vi "Test_Selection.vi"() -> ()   [LabVIEW 2017]
panel:
  out "File Transfer":u8
  in  "Recipe Download msg":string
  out "Exit":bool
  in  "Access Level":string
  out "Text Files":string[](array[string])
  out "Tests":string[](array[string])
  out "Paths":T1
  out "Rights":T2
  in  "Operator":string
  in  "Serial:":string
  in  "Part:":string
  in  "Test:":string
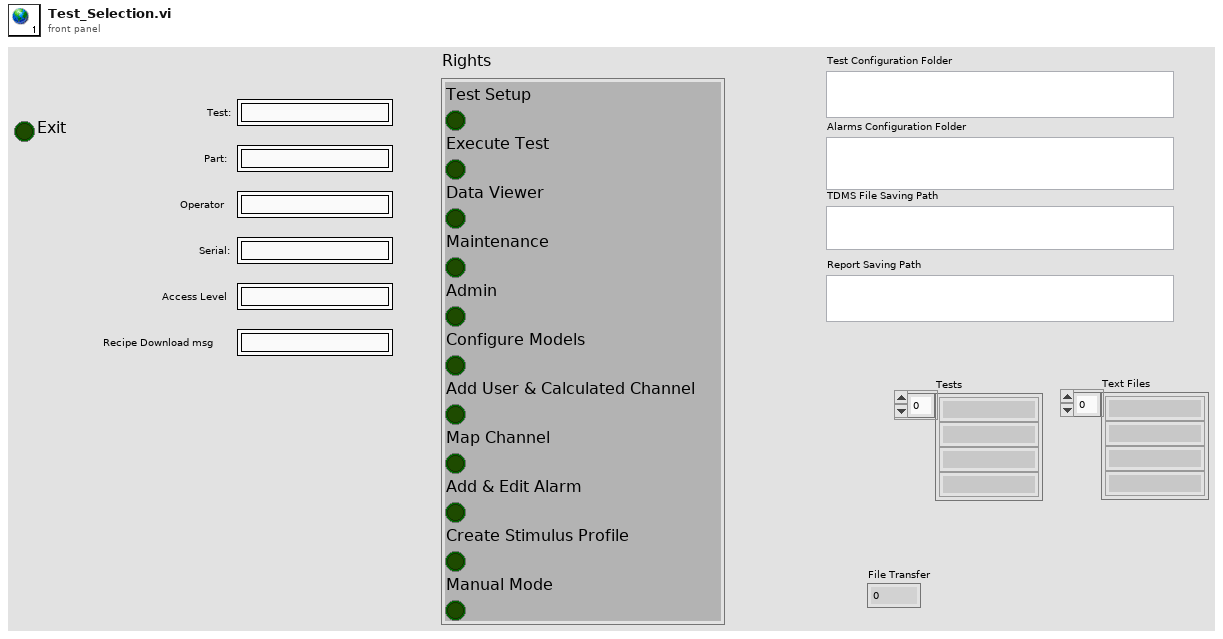
[diagram p1: front panel]
types:
  T1 = cluster{"Test Configuration Folder":path, "Alarms Configuration Folder":path, "TDMS File Saving Path":path, "Report Saving Path":path}
  T2 = cluster{"Test Setup":bool, "Execute Test":bool, "Data Viewer":bool, "Maintenance":bool, "Admin":bool, "Configure Models":bool, "Add User & Calculated Channel":bool, "Map Channel":bool, "Add & Edit Alarm":bool, "Create Stimulus Profile":bool, "Manual Mode":bool}
diagram:
